vi "Fdx Configure Board.vi"(7 "ExpertMode(ExpertMode)":T1 {"Expert1Mode" items=["FDX_EXPERT_MODE", "FDX_DISA_GHOST"]; "Expert2Mode" items=["FDX_EXPERT_MODE", "FDX_DISA_GHOST"]; "Expert3Mode" items=["FDX_EXPERT_MODE", "FDX_DISA_GHOST"]; "Expert4Mode" items=["FDX_EXPERT_MODE", "FDX_DISA_GHOST"]}, 8 "error in (no error)":errorcluster, 9 "PortSpeed (100Mbit)":T3 {"Port4SpeedIn" items=["FDX_100MBIT"=0, "FDX_10MBIT"=1, "FDX_AUTO_100MBIT"=2, "FDX_AUTO_10MBIT"=3, "FDX_1000MBIT"=5]; "Port3SpeedIn" items=["FDX_100MBIT"=0, "FDX_10MBIT"=1, "FDX_AUTO_100MBIT"=2, "FDX_AUTO_10MBIT"=3, "FDX_1000MBIT"=5]; "Port2SpeedIn" items=["FDX_100MBIT"=0, "FDX_10MBIT"=1, "FDX_AUTO_100MBIT"=2, "FDX_AUTO_10MBIT"=3, "FDX_1000MBIT"=5]; "Port1SpeedIn" items=["FDX_100MBIT"=0, "FDX_10MBIT"=1, "FDX_AUTO_100MBIT"=2, "FDX_AUTO_10MBIT"=3, "FDX_1000MBIT"=5]}, 10 "PortConfig (single)":T2 {"Port1ConfigIn" items=["FDX_SINGLE", "FDX_REDUNDANT"]; "Port2ConfigIn" items=["FDX_SINGLE", "FDX_REDUNDANT"]; "Port3ConfigIn" items=["FDX_SINGLE", "FDX_REDUNDANT"]; "Port4ConfigIn" items=["FDX_SINGLE", "FDX_REDUNDANT"]}, 11 "board index":u32) -> (0 "error out":errorcluster, 1 "timed out":bool, 2 "BSP Version Out":T4, 3 "Board Control Out":T5 {"SharedMemFree" format="%x"; "GlobalMemFree" format="%x"; "ExpertMode" items=["FDX_EXPERT_MODE", "FDX_DISA_GHOST"]; "PortGoodLink" items=["FDX_NO_LINK", "FDX_GOOD_LINK"]; "PortSpeed" items=["FDX_100MBIT", "FDX_10MBIT", "FDX_AUTO_100MBIT", "FDX_AUTO_10MBIT", "FDX_AUTO_ERROR", "FDX_1000MBIT"]; "PortConfig" items=["FDX_SINGLE", "FDX_REDUNDANT"]}, 4 "new config":bool)   [LabVIEW 2020, in "AIM664LV.lvlib"]
uses:
  AIM664LV.lvlib
  _controls/initialize_PortSpeed.ctl
  _controls/initialize_PortConfig.ctl
  _controls/initialize_ExpertMode.ctl
  _controls/hwEntry_actions.ctl
panel:
  in  "timeout ms (5000)":u32=5000
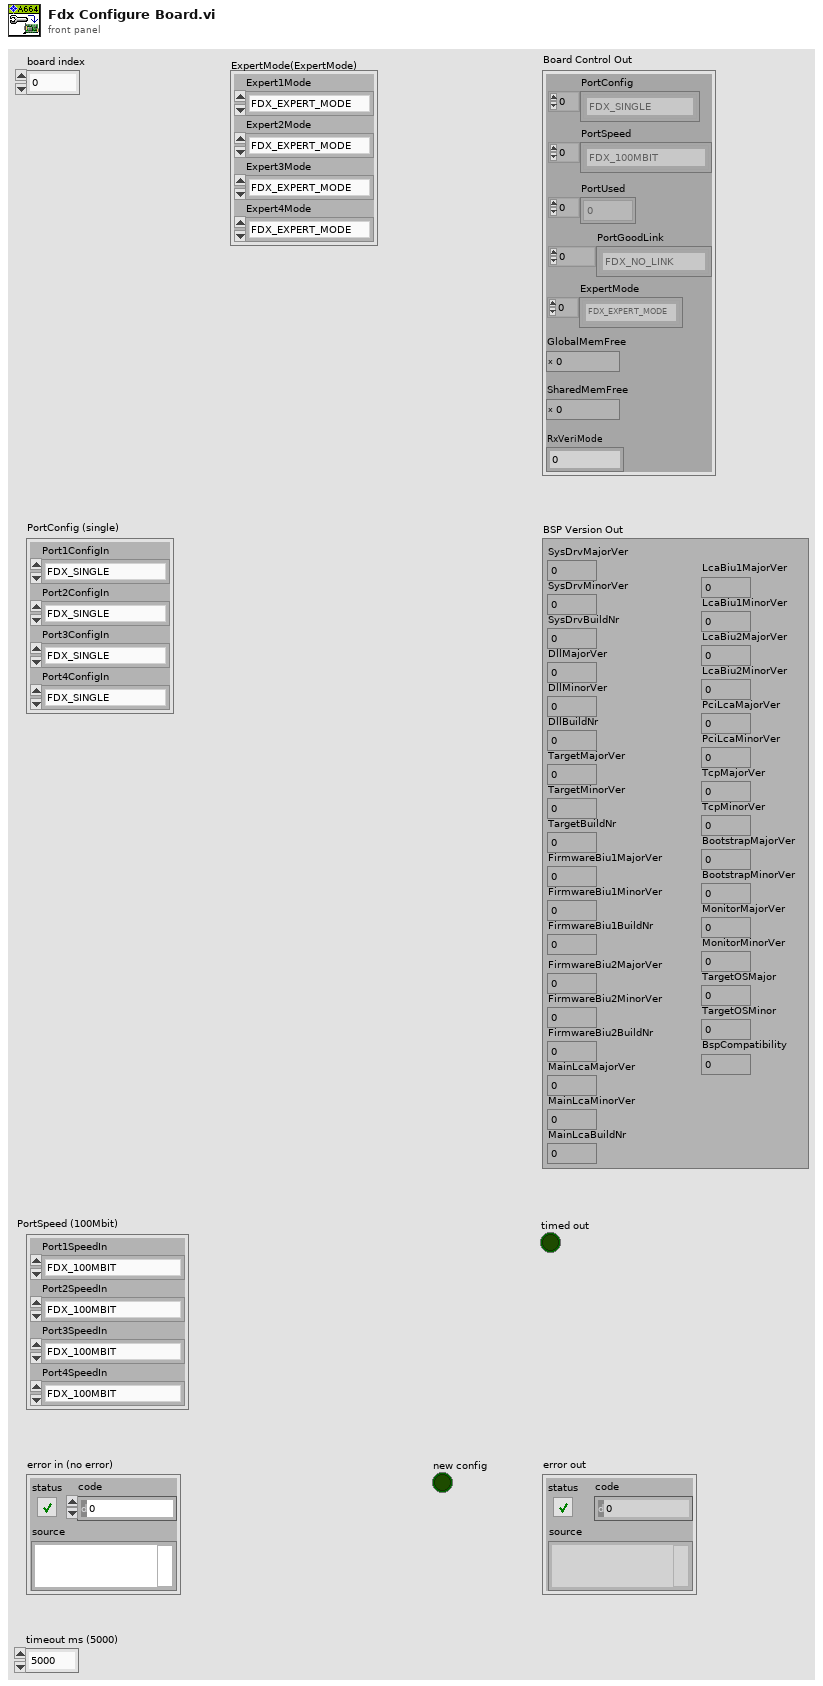
[diagram p1: front panel]
types:
  T1 = typedef "AIM664LV.lvlib/initialize_ExpertMode.ctl" = cluster{"Expert1Mode":u32, "Expert2Mode":u32, "Expert3Mode":u32, "Expert4Mode":u32}
  T2 = typedef "AIM664LV.lvlib/initialize_PortConfig.ctl" = cluster{"Port1ConfigIn":u32, "Port2ConfigIn":u32, "Port3ConfigIn":u32, "Port4ConfigIn":u32}
  T3 = typedef "AIM664LV.lvlib/initialize_PortSpeed.ctl" = cluster{"Port1SpeedIn":u32, "Port2SpeedIn":u32, "Port3SpeedIn":u32, "Port4SpeedIn":u32}
  T4 = cluster{"SysDrvMajorVer":u32, "SysDrvMinorVer":u32, "SysDrvBuildNr":u32, "DllMajorVer":u32, "DllMinorVer":u32, "DllBuildNr":u32, "TargetMajorVer":u32, "TargetMinorVer":u32, "TargetBuildNr":u32, "FirmwareBiu1MajorVer":u32, "FirmwareBiu1MinorVer":u32, "FirmwareBiu1BuildNr":u32, "FirmwareBiu2MajorVer":u32, "FirmwareBiu2MinorVer":u32, "FirmwareBiu2BuildNr":u32, "MainLcaMajorVer":u32, "MainLcaMinorVer":u32, "MainLcaBuildNr":u32, "LcaBiu1MajorVer":u32, "LcaBiu1MinorVer":u32, "LcaBiu2MajorVer":u32, "LcaBiu2MinorVer":u32, "PciLcaMajorVer":u32, "PciLcaMinorVer":u32, "TcpMajorVer":u32, "TcpMinorVer":u32, "BootstrapMajorVer":u32, "BootstrapMinorVer":u32, "MonitorMajorVer":u32, "MonitorMinorVer":u32, "TargetOSMajor":u32, "TargetOSMinor":u32, "BspCompatibility":u32}
  T5 = cluster{"PortConfig":u32[], "PortSpeed":u32[], "PortUsed":u32[], "PortGoodLink":u32[], "ExpertMode":u32[], "GlobalMemFree":u32, "SharedMemFree":u32, "RxVeriMode":u32}
  T6 = typedef "AIM664LV.lvlib/hwEntry_actions.ctl" = enum16{"Init Port", "Init Board", "Relase Port", "Release Board"}
  T7 = cluster{"Control":u32, "Port1ConfigIn":u32, "Port2ConfigIn":u32, "Port3ConfigIn":u32, "Port4ConfigIn":u32, "Port1SpeedIn":u32, "Port2SpeedIn":u32, "Port3SpeedIn":u32, "Port4SpeedIn":u32, "Expert1Mode":u32, "Expert2Mode":u32, "Expert3Mode":u32, "Expert4Mode":u32, "RxVeriModeIn":u32, "RxVeriData1":u32, "RxVeriData2":u32, "RxVeriData3":u32, "RxVeriData4":u32, "RxVeriData5":u32, "RxVeriData6":u32, "RxVeriData7":u32, "RxVeriData8":u32, "RxVeriMask1":u32, "RxVeriMask2":u32, "RxVeriMask3":u32, "RxVeriMask4":u32, "RxVeriMask5":u32, "RxVeriMask6":u32, "RxVeriMask7":u32, "RxVeriMask8":u32}
  T8 = typedef "AIM664LV.lvlib/port_configuration.ctl" = u32
  T9 = typedef "AIM664LV.lvlib/port_speed.ctl" = u32
  T10 = typedef "AIM664LV.lvlib/port_condition.ctl" = u32
  T11 = typedef "AIM664LV.lvlib/expert_mode.ctl" = u32
  T12 = cluster{"PortConfig":T8[], "PortSpeed":T9[], "PortUsed":u32[], "PortGoodLink":T10[], "ExpertMode":T11[], "GlobalMemFree":u32, "SharedMemFree":u32, "RxVeriMode":u32}
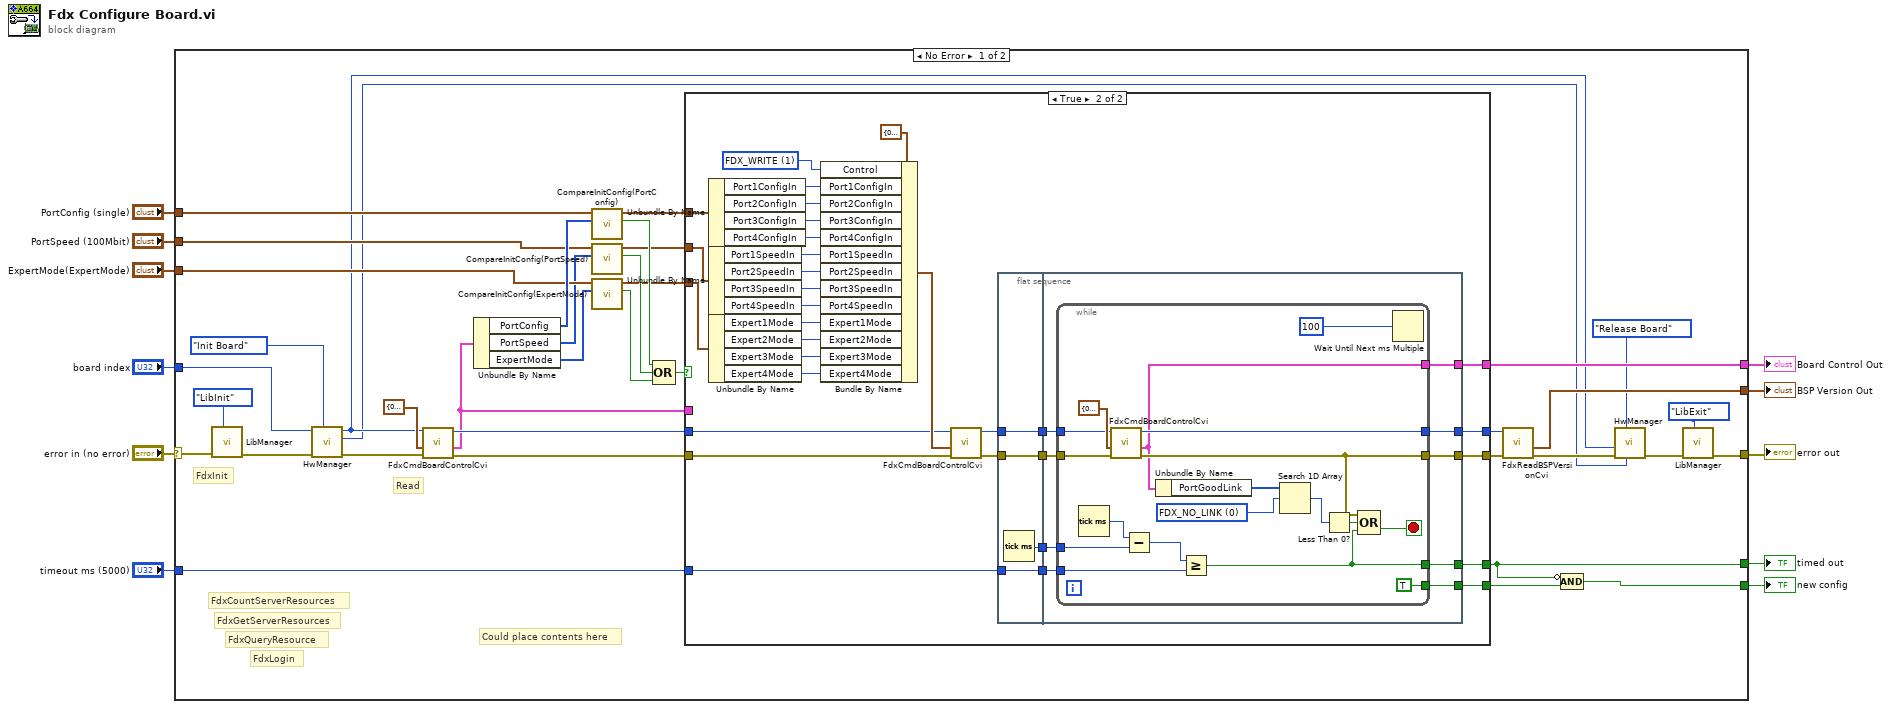
[diagram p0: block diagram]
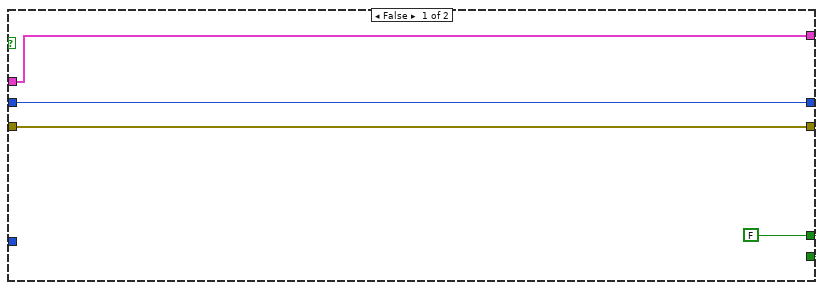
[diagram p2: hidden frame]
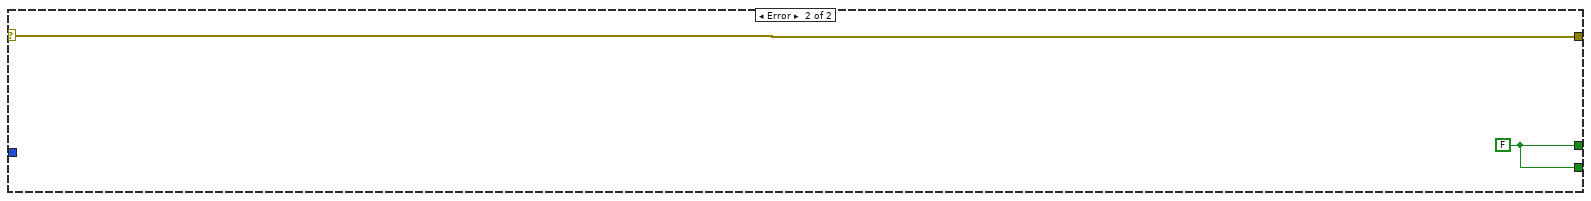
[diagram p3: hidden frame]
diagram:
  n1 = case shown="No Error" "error in (no error)" {
    selector: "error in (no error)" -> [w48 w118]
    tunnel: "board index" -> [w45 _]
    tunnel: [w44 _] -> w9
    tunnel: "ExpertMode(ExpertMode)" -> [w38 _]
    tunnel: "PortSpeed (100Mbit)" -> [w39 _]
    tunnel: "PortConfig (single)" -> [w41 _]
    tunnel: "timeout ms (5000)" -> [w28 _]
    tunnel: [w15 w117] -> w4
    tunnel: [w13 w118] -> w3
    tunnel: [w25 _] -> w2
    tunnel: [w16 w117] -> w1
    frame No Error {
      # "Read"
      # "Could place contents here"
      # "FdxLogin"
      # "FdxQueryResource"
      # "FdxGetServerResources"
      # "FdxCountServerResources"
      # "FdxInit"
      n2 = call "LibManager.vi"("action"=enum16{"LibInit", "LibExit"}."LibInit", "error in (no error)"=w48) -> ("error out"=w46:errorcluster)  [unwired: 7 in, 2 out]
      n3 = call "HwManager.vi"("action (Init)"=hwEntry_actions."Init Board", "error in (no error)"=w46, "board"=w45) -> ("error out"=w43:errorcluster, "InstrumentHandle_port out"=w18:u32, "InstrumentHandle_board out"=w19:u32)  [unwired: 4 in, 2 out]
      n4 = call "FdxCmdBoardControlCvi.vi"("error in"=w43, "BoardControlIn (read)"=T7 {"Control"=0, "Port1ConfigIn"=0, "Port2ConfigIn"=0, "Port3ConfigIn"=0, "Port4ConfigIn"=0, "Port1SpeedIn"=0, "Port2SpeedIn"=0, "Port3SpeedIn"=0, "Port4SpeedIn"=0, "Expert1Mode"=0, "Expert2Mode"=0, "Expert3Mode"=0, "Expert4Mode"=0, "RxVeriModeIn"=0, "RxVeriData1"=0, "RxVeriData2"=0, "RxVeriData3"=0, "RxVeriData4"=0, "RxVeriData5"=0, "RxVeriData6"=0, "RxVeriData7"=0, "RxVeriData8"=0, "RxVeriMask1"=0, "RxVeriMask2"=0, "RxVeriMask3"=0, "RxVeriMask4"=0, "RxVeriMask5"=0, "RxVeriMask6"=0, "RxVeriMask7"=0, "RxVeriMask8"=0} ("BoardControlIn"), "InstrumentHandle_board in"=w19) -> ("error out"=w32:errorcluster, "Board Control Out"=w27:T12, "InstrumentHandle_board out"=w30:u32)  [unwired: 6 in]
      n5 = Unbundle By Name(w27) -> ("PortConfig"=w40:T8[], "PortSpeed"=w36:T9[], "ExpertMode"=w37:T11[])
      n6 = call "CompareInitConfig(PortConfig).vi"("PortConfig - existing"=w40, "PortConfig - New"=w41) -> ("not equal"=w35:bool, "PortConfig - New out"=w24:T2)  [unwired: 8 in]
      n7 = call "CompareInitConfig(PortSpeed).vi"("PortSpeed - existing"=w36, "PortSpeed - new"=w39) -> ("not equal"=w34:bool, "PortSpeed - new out"=w23:T3)  [unwired: 8 in]
      n8 = call "CompareInitConfig(ExpertMode).vi"("ExpertMode - existing"=w37, "ExpertMode - new"=w38) -> ("not equal"=w33:bool, "ExpertMode - out"=w22:T1)  [unwired: 8 in]
      n9 = Compound Arithmetic op=OR(w35, w34, w33) -> (w31:bool)
      n10 = case shown="True" w31 {
        tunnel: w32 -> [w52 w81]
        tunnel: w30 -> [w53 w82]
        tunnel: [w52 w74] -> w29
        tunnel: w28 -> [_ w80]
        tunnel: w27 -> [w51 _]
        tunnel: [w50 w72] -> w15
        tunnel: [w53 w71] -> w26
        tunnel: [w51 w70] -> w25
        tunnel: w24 -> [_ w69]
        tunnel: w23 -> [_ w63]
        tunnel: w22 -> [_ w62]
        tunnel: [w50 w54] -> w17
        frame False {
          w50 = FALSE
        }
        frame True {
          w84 = u32 1 items=["FDX_READ", "FDX_WRITE"] ("Control")
          n11 = Unbundle By Name(w69) -> ("Port1ConfigIn"=w68:u32, "Port2ConfigIn"=w67:u32, "Port3ConfigIn"=w66:u32, "Port4ConfigIn"=w65:u32)
          n12 = Unbundle By Name(w63) -> ("Port1SpeedIn"=w64:u32, "Port2SpeedIn"=w61:u32, "Port3SpeedIn"=w60:u32, "Port4SpeedIn"=w59:u32)
          n13 = Unbundle By Name(w62) -> ("Expert1Mode"=w58:u32, "Expert2Mode"=w57:u32, "Expert3Mode"=w56:u32, "Expert4Mode"=w55:u32)
          n14 = Bundle By Name(cluster=T7 {"Control"=0, "Port1ConfigIn"=0, "Port2ConfigIn"=0, "Port3ConfigIn"=0, "Port4ConfigIn"=0, "Port1SpeedIn"=0, "Port2SpeedIn"=0, "Port3SpeedIn"=0, "Port4SpeedIn"=0, "Expert1Mode"=0, "Expert2Mode"=0, "Expert3Mode"=0, "Expert4Mode"=0, "RxVeriModeIn"=0, "RxVeriData1"=0, "RxVeriData2"=0, "RxVeriData3"=0, "RxVeriData4"=0, "RxVeriData5"=0, "RxVeriData6"=0, "RxVeriData7"=0, "RxVeriData8"=0, "RxVeriMask1"=0, "RxVeriMask2"=0, "RxVeriMask3"=0, "RxVeriMask4"=0, "RxVeriMask5"=0, "RxVeriMask6"=0, "RxVeriMask7"=0, "RxVeriMask8"=0} ("BoardControlIn"), "Control"=w84, "Port1ConfigIn"=w68, "Port2ConfigIn"=w67, "Port3ConfigIn"=w66, "Port4ConfigIn"=w65, "Port1SpeedIn"=w64, "Port2SpeedIn"=w61, "Port3SpeedIn"=w60, "Port4SpeedIn"=w59, "Expert1Mode"=w58, "Expert2Mode"=w57, "Expert3Mode"=w56, "Expert4Mode"=w55) -> (w83:T7)
          n15 = call "FdxCmdBoardControlCvi.vi"("error in"=w81, "BoardControlIn (read)"=w83, "InstrumentHandle_board in"=w82) -> ("error out"=w79:errorcluster, "InstrumentHandle_board out"=w78:u32)  [unwired: 6 in, 1 out]
          n16 = flat-sequence {
            tunnel: w78 -> [w87]
            tunnel: w79 -> [w88]
            tunnel: w80 -> [w89]
            tunnel: [w89] -> w77
            tunnel: [w88] -> w76
            tunnel: [w87] -> w75
            tunnel: [w86] -> w73
            tunnel: w77 -> [w98]
            tunnel: w76 -> [w97]
            tunnel: w75 -> [w96]
            tunnel: [w95] -> w74
            tunnel: w73 -> [w94]
            tunnel: [w93] -> w72
            tunnel: [w92] -> w71
            tunnel: [w91] -> w70
            tunnel: [w90] -> w54
            frame #0 {
              n17 = Tick Count (ms)() -> (millisecond timer value=w86:u32)
            }
            frame #1 {
              n18 = while {
                tunnel: w98 -> [w105]
                tunnel: w97 -> [w114]
                tunnel: w96 -> [w113]
                tunnel: [w103] -> w95
                tunnel: w94 -> [w107]
                tunnel: [w102] -> w93
                tunnel: [w101] -> w92
                tunnel: [w100] -> w91
                tunnel: [TRUE] -> w90
                stop <- w104 stop-if-true
                w111 = u32 0 items=["FDX_NO_LINK", "FDX_GOOD_LINK"]
                n19 = Tick Count (ms)() -> (millisecond timer value=w108:u32)
                n20 = call "FdxCmdBoardControlCvi.vi"("error in"=w114, "BoardControlIn (read)"=T7 {"Control"=0, "Port1ConfigIn"=0, "Port2ConfigIn"=0, "Port3ConfigIn"=0, "Port4ConfigIn"=0, "Port1SpeedIn"=0, "Port2SpeedIn"=0, "Port3SpeedIn"=0, "Port4SpeedIn"=0, "Expert1Mode"=0, "Expert2Mode"=0, "Expert3Mode"=0, "Expert4Mode"=0, "RxVeriModeIn"=0, "RxVeriData1"=0, "RxVeriData2"=0, "RxVeriData3"=0, "RxVeriData4"=0, "RxVeriData5"=0, "RxVeriData6"=0, "RxVeriData7"=0, "RxVeriData8"=0, "RxVeriMask1"=0, "RxVeriMask2"=0, "RxVeriMask3"=0, "RxVeriMask4"=0, "RxVeriMask5"=0, "RxVeriMask6"=0, "RxVeriMask7"=0, "RxVeriMask8"=0} ("BoardControlIn"), "InstrumentHandle_board in"=w113) -> ("error out"=w103:errorcluster, "Board Control Out"=w100:T12, "InstrumentHandle_board out"=w101:u32)  [unwired: 6 in]
                n21 = Subtract(x=w108, y=w107) -> (x-y=w106:u32)
                n22 = Unbundle By Name(w100) -> ("PortGoodLink"=w112:T10[])
                n23 = Greater Or Equal?(x=w106, y=w105) -> (x >= y?=w102:bool)
                n24 = Search 1D Array(1D array=w112, element=w111) -> (index of element=w109:i32)  [unwired: 1 in]
                n25 = Less Than 0?(x=w109) -> (x < 0?=w110:bool)
                n26 = Compound Arithmetic op=OR(w103, w110, w102) -> (w104:bool)
                n27 = Wait Until Next ms Multiple(millisecond multiple=u32 100) -> ()  [unwired: 1 out]
              }
            }
          }
        }
      }
      n28 = call "FdxReadBSPVersionCvi.vi"("error in"=w29, "InstrumentHandle_board in"=w26) -> ("error out"=w21:errorcluster, "BSP Version Out"=w44:T4)  [unwired: 7 in, 1 out]
      n29 = Compound Arithmetic op=AND(invert w15, w17) -> (w16:bool)
      n30 = call "HwManager.vi"("InstrumentHandle_port in"=w18, "action (Init)"=hwEntry_actions."Release Board", "error in (no error)"=w21, "InstrumentHandle_board in"=w19) -> ("error out"=w14:errorcluster)  [unwired: 3 in, 4 out]
      n31 = call "LibManager.vi"("action"=enum16{"LibInit", "LibExit"}."LibExit", "error in (no error)"=w14) -> ("error out"=w13:errorcluster)  [unwired: 7 in, 2 out]
    }
    frame Error {
      w117 = FALSE
    }
  }
  "error out" <- w3
  "Board Control Out" <- w2
  "BSP Version Out" <- w9
  "timed out" <- w4
  "new config" <- w1
